vi "5XY0.vi"(11 "Variables and Memory in":T1 {"GFX" format="%02x"}) -> (3 "Variables and Memory out":T1 {"GFX" format="%02x"})   [LabVIEW 2021]
uses:
  Controls/ClusterF.ctl
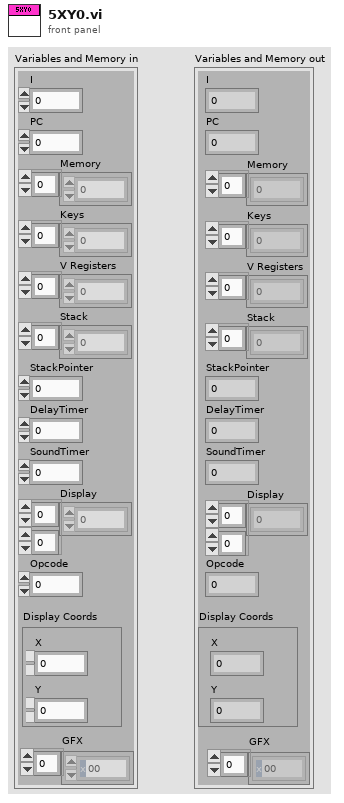
[diagram p1: front panel]
types:
  T1 = typedef "ClusterF.ctl" = cluster{"I":u16, "PC":u16, "Memory":u8[], "Keys":u8[], "V Registers":u8[], "Stack":u16[], "StackPointer":u16, "DelayTimer":u8, "SoundTimer":u8, "Display":u8[][], "Opcode":u16, "Display Coords":cluster{"X":u8, "Y":u8}, "GFX":u8[]}
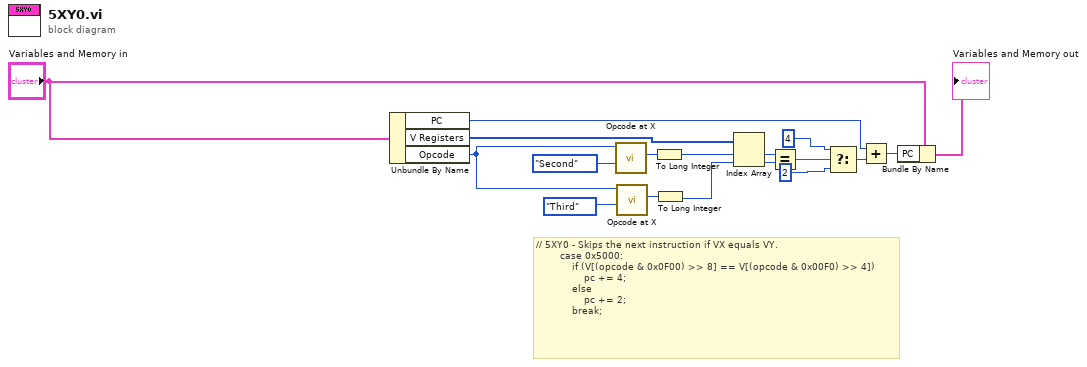
[diagram p0: block diagram]
diagram:
  # "// 5XY0 - Skips the next instruction if VX equals VY.\n        case 0x5000:\n            if (V[(opcode & 0x0F00) >> 8] == V[(opcode & 0x00F0) >> 4])\n                pc += 4;\n            else\n                pc += 2;\n            break;"
  n1 = Unbundle By Name("Variables and Memory in") -> ("PC"=w3:u16, "V Registers"=w18:u8[], "Opcode"=w7:u16)
  n2 = call "Opcode at X.vi"("X Position"=enum16{"First", "Second", "Third", "Fourth"}."Second", "Opcode"=w7) -> ("Opcode at X Position (U8)"=w10:u8)  [unwired: 9 in]
  n3 = call "Opcode at X.vi"("X Position"=enum16{"First", "Second", "Third", "Fourth"}."Third", "Opcode"=w7) -> ("Opcode at X Position (U8)"=w2:u8)  [unwired: 9 in]
  n4 = To Long Integer(number=w10) -> (32bit integer=w9:i32)
  n5 = To Long Integer(number=w2) -> (32bit integer=w16:i32)
  n6 = Index Array(array=w18, index #1=w9, index #2=w16) -> (element #1=w11:u8, element #2=w17:u8)
  n7 = Equal?(x=w11, y=w17) -> (x = y?=w15:bool)
  n8 = Select(t=u16 4 ("y"), s=w15, f=u16 2 ("y")) -> (s? t:f=w14:u16)
  n9 = Add(x=w3, y=w14) -> (x+y=w4:u16)
  n10 = Bundle By Name(cluster="Variables and Memory in", "PC"=w4) -> (→"Variables and Memory out":T1)
